vi "Scan to Next.vi"(9 "Indent":i32, 10 "Offset":i32, 11 "YAML":string="company: spacelift\ndomain:\n - devops\n - devsecops\ntutorial:\n  - yaml:\n      name: \"YAML Ain't Markup Language\"\n      type: awesome\n      born: 2001\n  - json:\n      name: JavaScript Object Notation\n      type: great\n      born: 2001\n  - xml:\n      name: Extensible Markup Language\n      type: good\n      born: 1996\nauthor: omkarbirade\npublished: true") -> (1 "Value Type":T1, 2 "Next":i32, 3 "Next Indent":i32)   [LabVIEW 2020, in "CDM-Config.lvlib" / "Config-YAML.lvclass"]
uses:
  Config-YAML.lvclass
  Config-YAML.lvclass/Config-YAML.ctl
  Value Type.ctl
  CDM-Config.lvlib
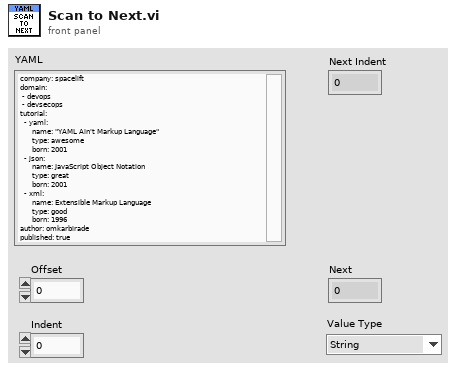
[diagram p1: front panel]
types:
  T1 = typedef "CDM-Config.lvlib/Value Type.ctl" = enum16{"String", "Number", "Bool", "Object", "Array"}
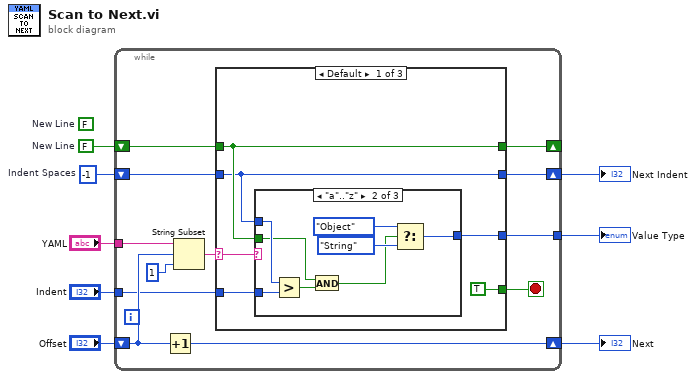
[diagram p0: block diagram]
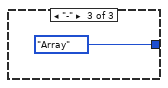
[diagram p3: hidden frame]
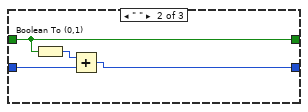
[diagram p4: hidden frame]
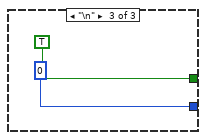
[diagram p5: hidden frame]
diagram:
  (unwired) FALSE  # New Line
  w5 = -1  # Indent Spaces
  w6 = FALSE  # New Line
  n1 = while {
    shift-right: [w12] -> w3
    shift-left: "Offset" -> [w16]
    tunnel: "YAML" -> [w20]
    shift-right: [w15] -> _
    shift-left: w6 -> [w17]
    shift-right: [w13] -> w4
    shift-left: w5 -> [w14]
    tunnel: [w11] -> w2
    tunnel: "Indent" -> [w9]
    stop <- w10 stop-if-true
    n2 = Increment(x=w16) -> (x+1=w12:i32)
    n3 = String Subset(string=w20, offset (0)=w16, length (rest)=1 ("length (rest)")) -> (substring=w18:string)
    n4 = case shown="Default" w18 {
      selector: w18 -> [w26 _ _]
      tunnel: w17 -> [w23 w39 _]
      tunnel: [w23 w39 TRUE] -> w15
      tunnel: w14 -> [w21 w38 _]
      tunnel: [w21 w36 0] -> w13
      tunnel: [w25 _ _] -> w11
      tunnel: [TRUE _ _] -> w10
      tunnel: w9 -> [w22 _ _]
      frame Default {
        n5 = case shown="\"a\"..\"z\"" w26 {
          tunnel: [_ w28 Value_Type."Array" ("Value Type")] -> w25
          tunnel: w23 -> [_ w31 _]
          tunnel: w22 -> [_ w34 _]
          tunnel: w21 -> [_ w33 _]
          frame Default {
          }
          frame "a".."z" {
            n6 = Greater?(x=w33, y=w34) -> (0:w32:bool)
            n7 = And(x=w31, y=w32) -> (x .and. y?=w27:bool)
            n8 = Select(t=Value_Type."Object" ("Value Type"), s=w27, f=Value_Type."String" ("Value Type")) -> (s? t:f=w28:T1)
          }
          frame "-" {
          }
        }
      }
      frame " " {
        n9 = Boolean To (0,1)(Boolean=w39) -> (0, 1=w37:i16)
        n10 = Add(x=w37, y=w38) -> (x+y=w36:i32)
      }
      frame "\n" {
      }
    }
  }
  "Next" <- w3
  "Next Indent" <- w4
  "Value Type" <- w2
